vi "set_params.vi"(8 "error in (no error)":errorcluster caption="entrée d'erreur (pas d'erreur)", 11 "LatentDirichletAllocation.lvclass":refnum<class "LatentDirichletAllocation.lvclass">) -> (0 "error out":errorcluster caption="sortie d'erreur", 3 "LatentDirichletAllocation.lvclass 2":refnum<class "LatentDirichletAllocation.lvclass">)   [LabVIEW 2020, in "LatentDirichletAllocation.lvclass"]
uses:
  LatentDirichletAllocation.lvclass
  LatentDirichletAllocation.lvclass/LatentDirichletAllocation.ctl
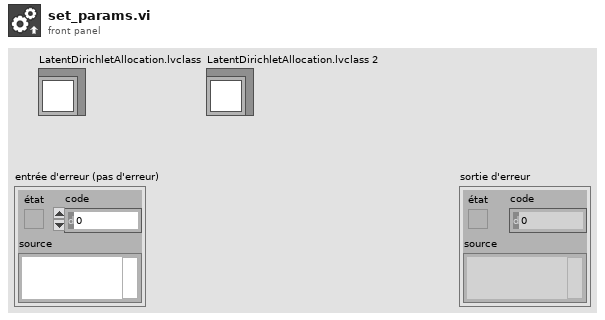
[diagram p1: front panel]
types:
  T1 = typedef "latent_dirichlet_allocation_params.ctl" = cluster{"n_components":dbl, "doc_topic_prior":cluster{"doc_topic_prior_type":string, "doc_topic_prior_float":dbl}, "topic_word_prior":cluster{"topic_word_prior_type":string, "topic_word_prior_float":dbl}, "learning_method":string, "learning_decay":dbl, "learning_offset":dbl, "max_iter":dbl, "batch_size":dbl, "evaluate_every":dbl, "total_samples":i32, "perp_tol":dbl, "mean_change_tol":dbl, "max_doc_update_iter":dbl, "n_jobs":dbl, "verbose":dbl, "random_state":dbl}
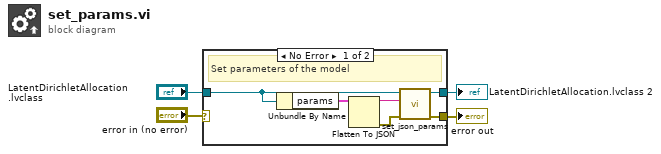
[diagram p0: block diagram]
diagram:
  n1 = case shown="No Error" "error in (no error)" {
    selector: "error in (no error)" -> [_ w12]
    tunnel: [w7 w12] -> w3
    tunnel: [w8 w11] -> w1
    tunnel: "LatentDirichletAllocation.lvclass" -> [w5 w11]
    frame No Error {
      # "Set parameters of the model"
      n2 = Unbundle By Name(w5) -> ("params"=w10:T1)
      n3 = Flatten To JSON(anything=w10) -> (JSON string=w9:string, 11:w6:errorcluster)  [unwired: 2 in]
      n4 = call-dynamic "set_json_params.vi"("error in (no error)"=w6, "params"=w9, "Model en entrée"=w5) -> ("error out"=w7:errorcluster, "Model en sortie"=w8:refnum<class "LatentDirichletAllocation.lvclass">)  [unwired: 7 in]
    }
    frame Error {
    }
  }
  "error out" <- w3
  "LatentDirichletAllocation.lvclass 2" <- w1
